vi "Get Process.vi"(8 "error in (no error)":errorcluster, 10 "Process Name":string, 11 "Rig In":refnum<class "Application.lvclass">) -> (0 "error out":errorcluster, 2 "App Process":refnum<class "Process.lvclass">, 3 "Rig Out":refnum<class "Application.lvclass">)   [LabVIEW 2020, in "Application.lvclass"]
doc: "Get a specific process by name. A good pattern for using this VI is to wrap it with a string constant fed into the Process Name input and cast the received process to the expected process class. This pattern makes changing the class or the name easy as there is only one this single location where it is specified."
uses:
  Application.lvclass
  C:/Users/anton/Documents/GitHub/Triarc-Framework/source/Framework/Process/Process.lvclass
  Process/Process.lvclass
  Process/Process.lvclass/Process.ctl
  Application.lvclass/Application.ctl
  <vilib>/Utility/error.llb/Clear Errors.vi
  Process/Private/SubVIs/Enqueue Request Message.vi
  <vilib>/Utility/error.llb/Error Cluster From Error Code.vi
  Process/Private/SubVIs/Wait for Response Message.vi
  <vilib>/ErrorRing/Error Ring.xnode
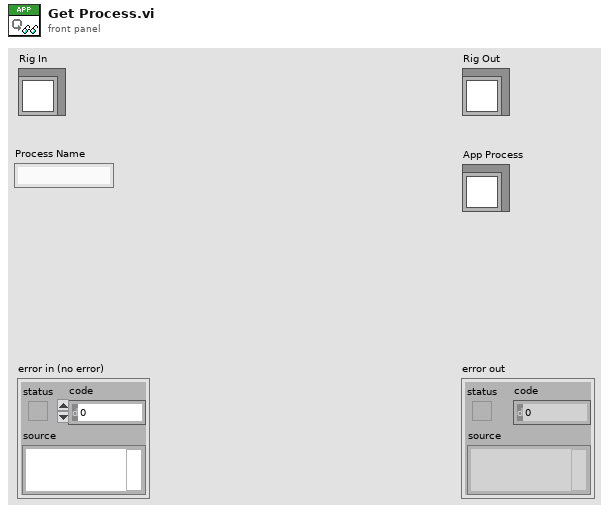
[diagram p1: front panel]
types:
  T1 = typedef "Process.lvclass/Lifecycle State.ctl" = enum16{"Uninitialized", "Initialized", "Started", "Running", "Stopped", "Finished"}
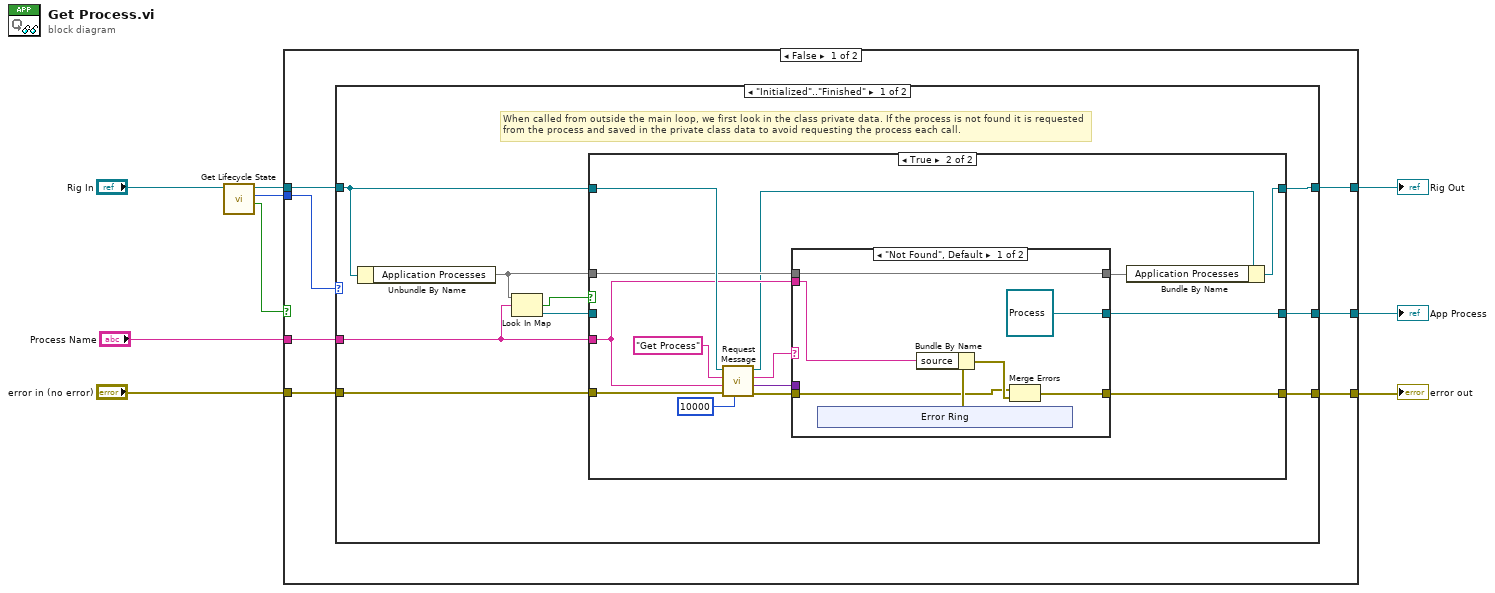
[diagram p0: block diagram]
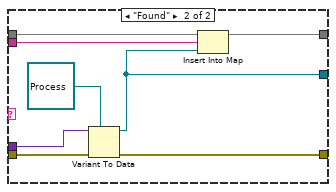
[diagram p3: hidden frame]
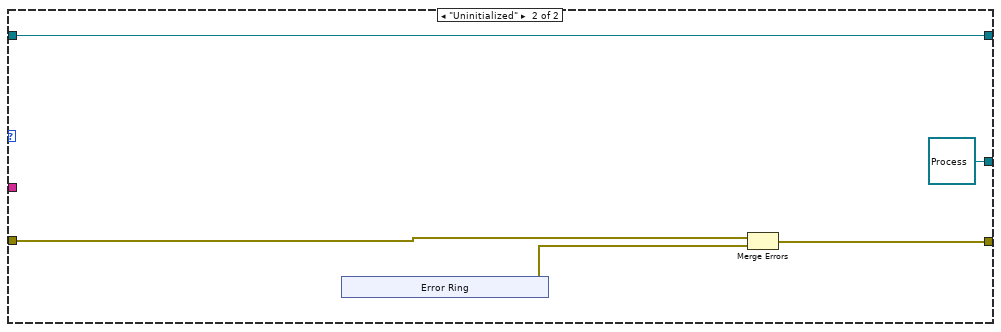
[diagram p4: hidden frame]
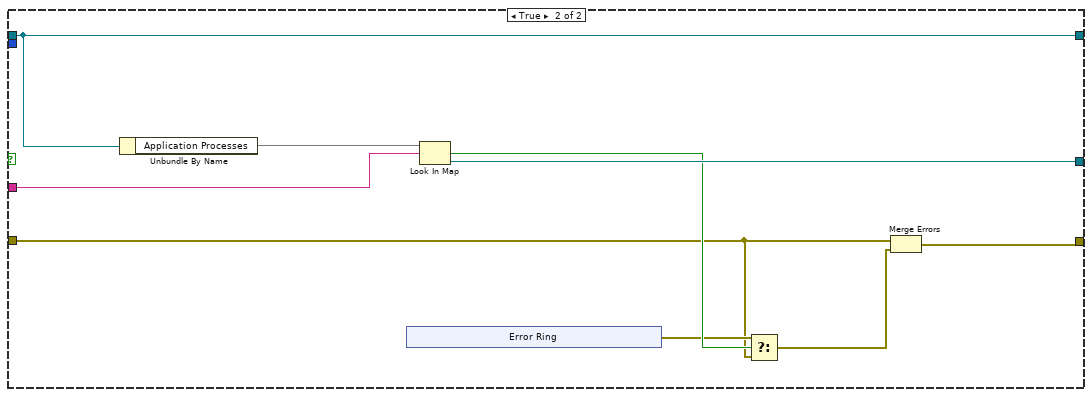
[diagram p5: hidden frame]
diagram:
  n1 = call "Get Lifecycle State.vi"("Process In"="Rig In") -> ("In Process Loop?"=w1:bool, "Lifecycle State"=w2:T1, "Process Out"=w3:refnum<class "Application.lvclass">)  [unwired: 7 in, 1 out]
  n2 = case shown="False" w1 {
    tunnel: "error in (no error)" -> [w16 w74]
    tunnel: "Process Name" -> [w15 w78]
    tunnel: [w14 w77] -> w6
    tunnel: [w13 w71] -> w5
    tunnel: [w12 w72] -> w4
    tunnel: w3 -> [w11 w71]
    tunnel: w2 -> [w10 _]
    frame False {
      n3 = case shown="\"Initialized\"..\"Finished\"" w10 {
        tunnel: [w18 w64] -> w12
        tunnel: [w19 refnum<class "Process.lvclass"> refnum ("Rig Process")] -> w14
        tunnel: w15 -> [w22 _]
        tunnel: [w20 w66] -> w13
        tunnel: w11 -> [w23 w66]
        tunnel: w16 -> [w21 w65]
        frame "Initialized".."Finished" {
          # "When called from outside the main loop, we first look in the class private data. If the process is not found it is requested from the process and saved in the private class data to avoid requesting the process each call."
          n4 = Unbundle By Name(w23) -> ("Application Processes"=w24:map{string, refnum<class "Process.lvclass">})
          n5 = Look In Map(map=w24, key=w22) -> (key not found?=w17:bool, value=w25:refnum<class "Process.lvclass">)  [unwired: 1 in]
          n6 = case shown="True" w17 {
            tunnel: [w27 w38] -> w18
            tunnel: [w28 w37] -> w19
            tunnel: w21 -> [w27 w36]
            tunnel: w23 -> [w26 w34]
            tunnel: w22 -> [_ w32]
            tunnel: w25 -> [w28 _]
            tunnel: w24 -> [_ w33]
            tunnel: [w26 w29] -> w20
            frame False {
              # "Or we have not started process"
              # "Or we are in process loop"
              # "Process has been requested before and is found in current object"
            }
            frame True {
              n7 = call "Request Message.vi"("timeout in ms (-1)"=10000, "error in (no error)"=w36, "Request Message Data"=w32, "Request Message"="Get Process", "Process In"=w34) -> ("error out"=w42:errorcluster, "Response Message Data"=w40:variant, "Response Message"=w35:string, "Process Out"=w31:refnum<class "Application.lvclass">)  [unwired: 2 in, 1 out]
              n8 = case shown="\"Not Found\", Default" w35 {
                tunnel: w42 -> [w43 w61]
                tunnel: w40 -> [_ w60]
                tunnel: [w44 w58] -> w38
                tunnel: [refnum<class "Process.lvclass"> refnum ("Rig Process") w54] -> w37
                tunnel: w33 -> [w48 w57]
                tunnel: w32 -> [w45 w56]
                tunnel: [w48 w55] -> w30
                frame "Not Found", Default {
                  n9 = xnode "Error Ring"() -> ("error out"=w47:errorcluster)
                  n10 = Bundle By Name(cluster=w47, "source"=w45) -> (w46:errorcluster)
                  n11 = Merge Errors(w43, w46) -> (w44:errorcluster)
                }
                frame "Found" {
                  n12 = Variant To Data(error in=w61, type=refnum<class "Process.lvclass"> refnum ("Rig Process"), Variant=w60) -> (data=w54:refnum<class "Process.lvclass">, error out=w58:errorcluster)
                  n13 = Insert Into Map(map in=w57, key=w56, value=w54) -> (map out=w55:map{string, refnum<class "Process.lvclass">})  [unwired: 2 out]
                }
              }
              n14 = Bundle By Name(cluster=w31, "Application Processes"=w30) -> (w29:refnum<class "Application.lvclass">)
            }
          }
        }
        frame "Uninitialized" {
          n15 = xnode "Error Ring"() -> ("error out"=w62:errorcluster)
          n16 = Merge Errors(w65, w62) -> (w64:errorcluster)
        }
      }
    }
    frame True {
      n17 = Unbundle By Name(w71) -> ("Application Processes"=w79:map{string, refnum<class "Process.lvclass">})
      n18 = xnode "Error Ring"() -> ("error out"=w75:errorcluster)
      n19 = Look In Map(map=w79, key=w78) -> (key not found?=w76:bool, value=w77:refnum<class "Process.lvclass">)  [unwired: 1 in]
      n20 = Select(t=w75, s=w76, f=w74) -> (s? t:f=w73:errorcluster)
      n21 = Merge Errors(w74, w73) -> (w72:errorcluster)
    }
  }
  "error out" <- w4
  "Rig Out" <- w5
  "App Process" <- w6
